vi "GetPluginType.vi"(0 "Instrument Modules In New":T1=[{"PluginSelection"=4, "ConfigDialog"=FALSE}], 1 "reference":refnum<vi>, 5 "Instrument Modules In Old":T1=[{"PluginSelection"=4, "ConfigDialog"=FALSE}], 7 "INIFilePaths":path[](array[path]), 9 "Compare? (F)":bool, 11 "ErrorArray In":errorcluster[](array[cluster]), 12 "Priority (2)":u8=2, 13 "Severity (Critical)":string="Critical") -> (3 "PluginTypes":string[](array[string]), 4 "Instrument Modules New Out":T1=[{"PluginSelection"=4, "ConfigDialog"=FALSE}], 6 "Instrument Modules Old Out":T1=[{"PluginSelection"=4, "ConfigDialog"=FALSE}], 10 "PluginSelection Changed?":bool, 15 "ErrorArray Out":errorcluster[](array[cluster]))   [LabVIEW 2018]
doc: "Extracts the plugin type from the configuration file."
uses:
  Framework/InstrumentModulesControl.ctl
  <vilib>/Utility/config.llb/Read Key (String).vi
  <vilib>/Utility/error.llb/Error Cluster From Error Code.vi
  <vilib>/ErrorRing/Error Ring.xnode
  LV_Ini/Ini_lib.lvlib
  <userlib>/NIST/NISTErrorLib/NISTErrorLib.lvlib
  <vilib>/Utility/config.llb/NI_LVConfig.lvlib
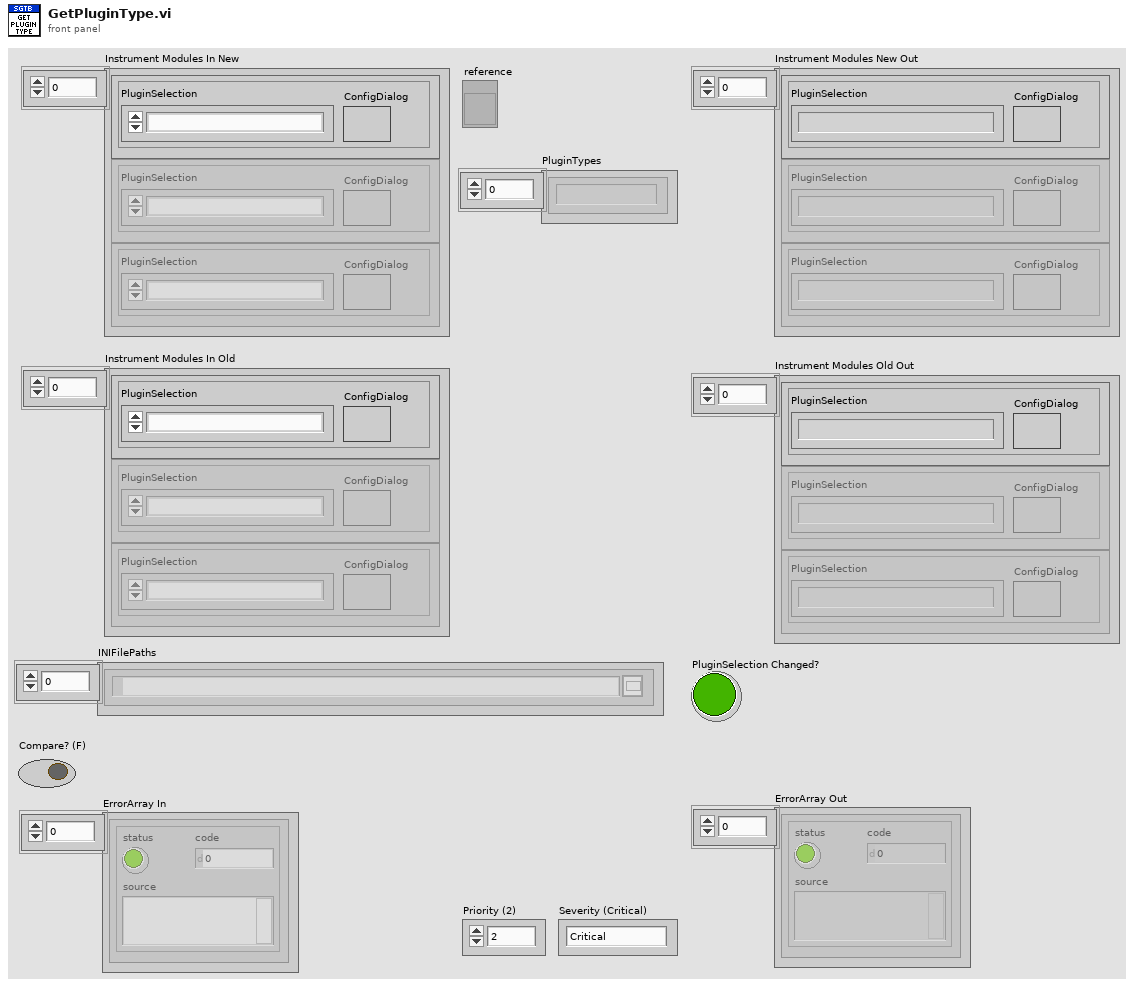
[diagram p1: front panel]
types:
  T1 = typedef "InstrumentModulesControl.ctl" = cluster{"PluginSelection":u16, "ConfigDialog":bool}[]
  T2 = typedef "NI_LVConfig.lvlib/Config Data RefNum.ctl" = refnum<k1>
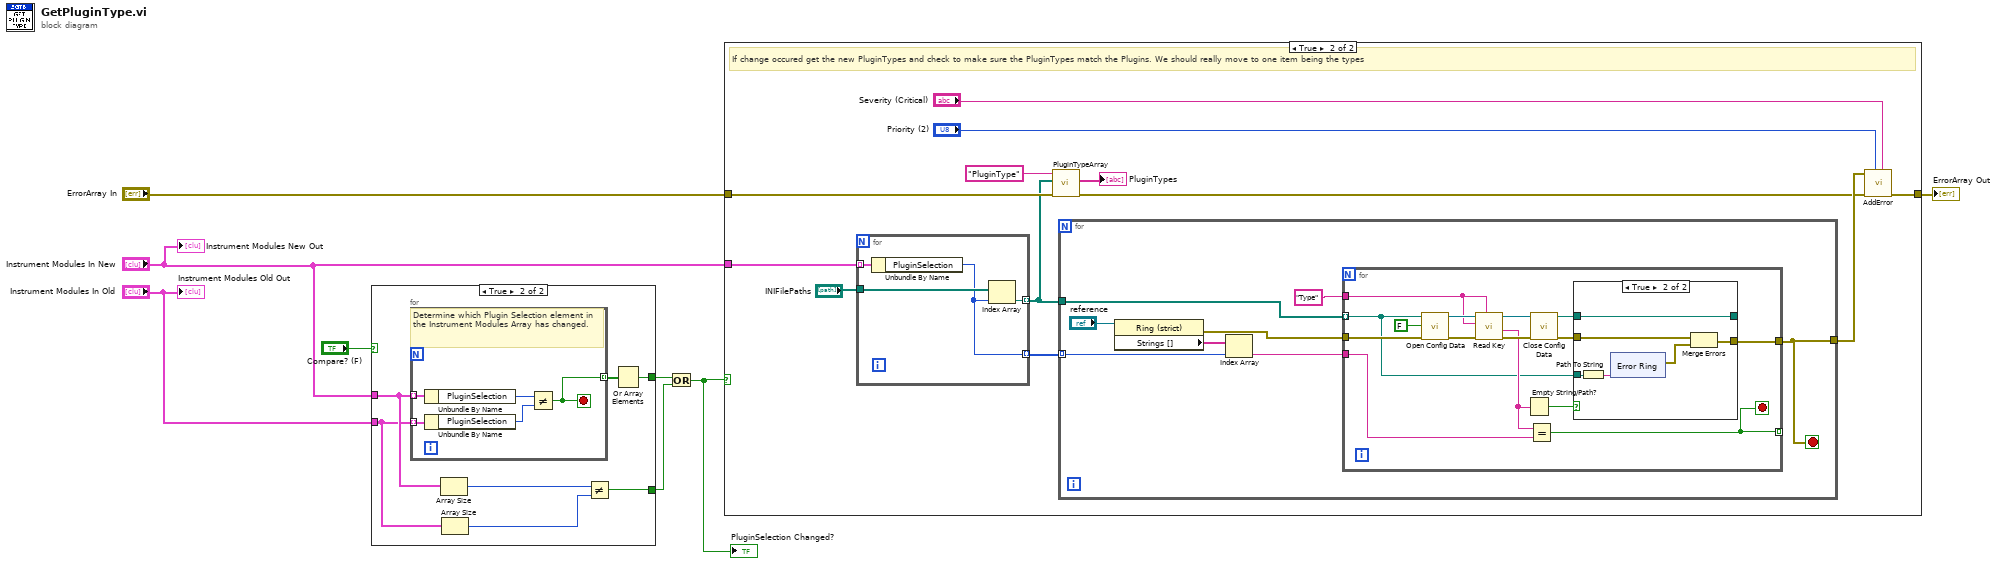
[diagram p0: block diagram]
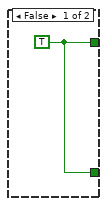
[diagram p2: hidden frame]
diagram:
  n1 = case shown="True" "Compare? (F)" {
    tunnel: "Instrument Modules In New" -> [_ w13]
    tunnel: "Instrument Modules In Old" -> [_ w12]
    tunnel: [w9 w15] -> w3
    tunnel: [w9 w14] -> w1
    frame False {
      w9 = TRUE
    }
    frame True {
      n2 = for {
        tunnel: w12 -> [w21] mode=indexing
        tunnel: w13 -> [w20] mode=indexing
        tunnel: [w17] -> w16 mode=indexing
        stop <- w17 stop-if-true
        # "Determine which Plugin Selection element in the Instrument Modules Array has changed."
        n3 = Unbundle By Name(w20) -> ("PluginSelection"=w19:u16)
        n4 = Unbundle By Name(w21) -> ("PluginSelection"=w18:u16)
        n5 = Not Equal?(x=w19, y=w18) -> (x != y?=w17:bool)
      }
      n6 = Array Size(array=w13) -> (size(s)=w10:i32)
      n7 = Array Size(array=w12) -> (size(s)=w11:i32)
      n8 = Not Equal?(x=w10, y=w11) -> (x != y?=w14:bool)
      n9 = Or Array Elements(Boolean array=w16) -> (logical OR=w15:bool)
    }
  }
  n10 = Or(x=w3, y=w1) -> (x .or. y?=w2:bool)
  "PluginSelection Changed?" <- w2
  n11 = case shown="True" w2 {
    tunnel: "ErrorArray In" -> [w22 w33]
    tunnel: "Instrument Modules In New" -> [_ w32]
    tunnel: [w22 w29] -> w7
    frame False {
      # "If no change occured do nothing."
    }
    frame True {
      # "If change occured get the new PluginTypes and check to make sure the PluginTypes match the Plugins. We should really move to one item being the types"
      n12 = for {
        tunnel: w32 -> [w38] mode=indexing
        tunnel: "INIFilePaths" -> [w37]
        tunnel: [w36] -> w27 mode=indexing
        tunnel: [w35] -> w28 mode=indexing
        n13 = Unbundle By Name(w38) -> ("PluginSelection"=w35:u16)
        n14 = Index Array(array=w37, index=w35) -> (element=w36:path)
      }
      n15 = call "PluginTypeArray.vi"("ErrorArray Out in"=w33, "INIFilePaths"=w27, "section"="PluginType") -> ("ErrorArray Out out"=w30:errorcluster[], "PluginTypes"=→"PluginTypes":string[])  [unwired: 6 in, 1 out]
      n16 = for {
        tunnel: [w43] -> w31
        tunnel: w28 -> [w44] mode=indexing
        tunnel: w27 -> [w42]
        stop <- w43 stop-if-true
        n17 = property class="Ring (strict)"(reference="reference") -> (error out=w41:errorcluster, "Strings []"=w46:string[])  [unwired: 1 in, 1 out]
        n18 = Index Array(array=w46, index=w44) -> (element=w40:string)
        n19 = for {
          tunnel: w42 -> [w47] mode=indexing
          tunnel: "Type" ("section") -> [w54]
          tunnel: w40 -> [w49]
          tunnel: [w52] -> w43
          tunnel: w41 -> [w51]
          tunnel: [w48] -> _ mode=indexing
          stop <- w48 stop-if-true
          n20 = call <vilib>:"Open Config Data.vi"("error in (no error)"=w51, "create file if necessary (T)"=FALSE, "configuration file path"=w47) -> ("error out"=w60:errorcluster, "refnum"=w59:T2)  [unwired: 6 in, 1 out]
          n21 = call-poly <vilib>:"Read Key.vi"("section"=w54, "error in (no error)"=w60, "key"=w54, "refnum"=w59) -> ("error out"=w57:errorcluster, "value"=w50:string, "refnum out"=w58:T2)  [unwired: 4 in, 1 out]
          n22 = Empty String/Path?(string/path=w50) -> (empty?=w56:bool)
          n23 = Equal?(x=w50, y=w49) -> (x = y?=w48:bool)
          n24 = call <vilib>:"Close Config Data.vi"("error in (no error)"=w57, "refnum"=w58) -> ("error out"=w55:errorcluster, "file path"=w53:path)  [unwired: 8 in]
          n25 = case shown="True" w56 {
            tunnel: w55 -> [w63 w68]
            tunnel: [w63 w67] -> w52
            tunnel: w47 -> [_ w65]
            tunnel: w53 -> [w62 w64]
            tunnel: [w62 w64] -> _
            frame False {
            }
            frame True {
              n26 = Path To String(path=w65) -> (string=w66:string)
              n27 = xnode "Error Ring"("parameter 0"=w66) -> ("error out"=w69:errorcluster)
              n28 = Merge Errors(w68, w69) -> (w67:errorcluster)
            }
          }
        }
      }
      n29 = call <userlib>:"AddError.vi"("Severity"="Severity (Critical)", "Priority"="Priority (2)", "ErrorArray In"=w30, "error in (no error)"=w31) -> ("ErrorArray Out"=w29:errorcluster[])  [unwired: 6 in, 1 out]
    }
  }
  "ErrorArray Out" <- w7
  "Instrument Modules New Out" <- "Instrument Modules In New"
  "Instrument Modules Old Out" <- "Instrument Modules In Old"
